vi "Determine Warnings.vi"(8 "error in (no error)":errorcluster, 9 "Min Temp":dbl, 10 "Max Temp":dbl, 11 "Current Temp":dbl) -> (0 "error out":errorcluster, 2 "Warning?":bool, 3 "Warning Text":string)   [LabVIEW 2014]
panel:
  # "You must create a portion of a larger project. The lead developer gives you the inputs of the VI, the\nalgorithm, and the expected outputs. Create and document a VI based on the given design."
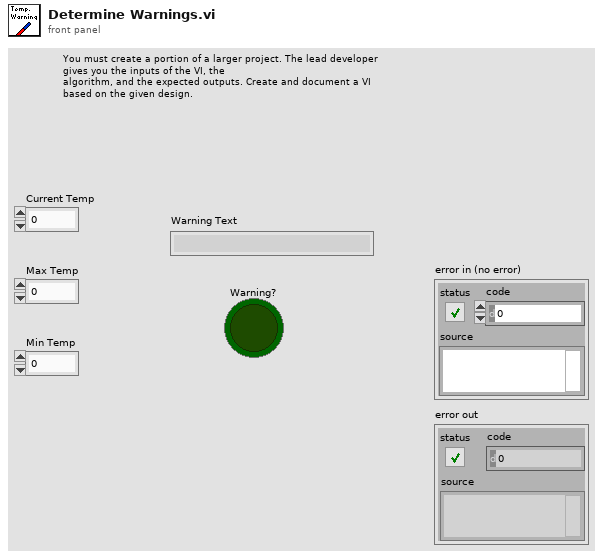
[diagram p1: front panel]
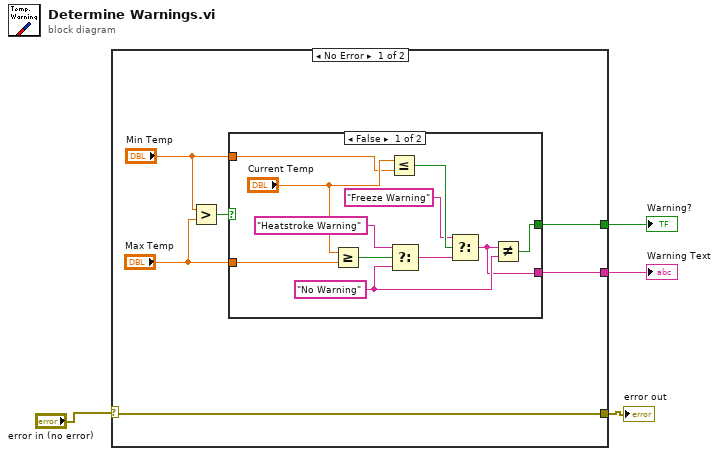
[diagram p0: block diagram]
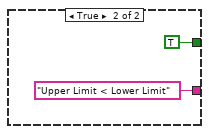
[diagram p2: hidden frame]
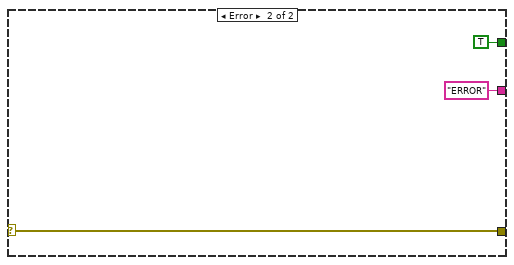
[diagram p3: hidden frame]
diagram:
  n1 = case shown="No Error" "error in (no error)" {
    selector: "error in (no error)" -> [w5 w24]
    tunnel: [w10 "ERROR"] -> w4
    tunnel: [w9 TRUE] -> w3
    tunnel: [w5 w24] -> w1
    frame No Error {
      n2 = Greater?(x="Min Temp", y="Max Temp") -> (0:w6:bool)
      n3 = case shown="False" w6 {
        tunnel: [w14 "Upper Limit < Lower Limit"] -> w10
        tunnel: [w13 TRUE] -> w9
        tunnel: "Max Temp" -> [w12 _]
        tunnel: "Min Temp" -> [w11 _]
        frame False {
          w20 = "No Warning"
          n4 = Greater Or Equal?(x="Current Temp", y=w12) -> (x >= y?=w15:bool)
          n5 = Less Or Equal?(x="Current Temp", y=w11) -> (x <= y?=w19:bool)
          n6 = Select(t="Heatstroke Warning", s=w15, f=w20) -> (s? t:f=w18:string)
          n7 = Select(t="Freeze Warning", s=w19, f=w18) -> (s? t:f=w14:string)
          n8 = Not Equal?(x=w14, y=w20) -> (x != y?=w13:bool)
        }
        frame True {
        }
      }
    }
    frame Error {
    }
  }
  "Warning?" <- w3
  "Warning Text" <- w4
  "error out" <- w1
